vi "Get DVR From Class.vi"(8 "error in (no error)":errorcluster, 10 "Path In":path, 11 "TX Speed.lvclass In":refnum<class "TX Speed.lvclass">) -> (0 "error out":errorcluster, 2 "Class DVR":refnum<data-value>, 3 "TX Speed.lvclass Out":refnum<class "TX Speed.lvclass">)   [LabVIEW 2020, in "TX Speed.lvclass"]
uses:
  TX Speed.lvclass
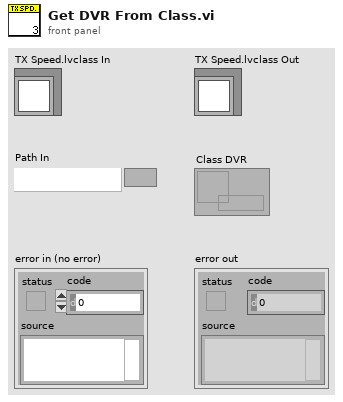
[diagram p1: front panel]
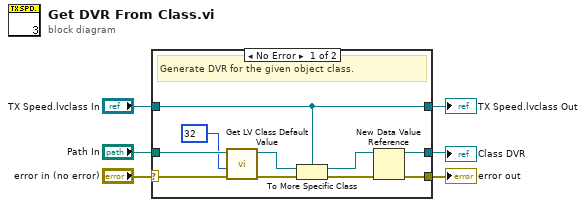
[diagram p0: block diagram]
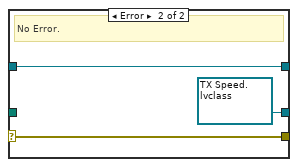
[diagram p2: hidden frame]
diagram:
  n1 = case shown="No Error" "error in (no error)" {
    selector: "error in (no error)" -> [w13 w19]
    tunnel: [w16 w19] -> w5
    tunnel: [w14 w18] -> w2
    tunnel: "TX Speed.lvclass In" -> [w14 w18]
    tunnel: "Path In" -> [w11 _]
    tunnel: [w8 refnum<data-value> refnum ("data value reference")] -> w1
    frame No Error {
      # "Generate DVR for the given object class."
      n2 = call <vilib>:"Get LV Class Default Value.vi"("error in (no error)"=w13, "options"=u32 32, "class path"=w11) -> ("error out"=w12:errorcluster, "object"=w10:refnum<class>)  [unwired: 7 in]
      n3 = To More Specific Class(target class=w14, reference=w10, error in=w12) -> (specific class reference=w9:refnum<class "TX Speed.lvclass">, error out=w15:errorcluster)
      n4 = New Data Value Reference(data value=w9, error in=w15) -> (data value reference=w8:refnum<data-value>, error out=w16:errorcluster)
    }
    frame Error {
      # "No Error."
    }
  }
  "Class DVR" <- w1
  "error out" <- w5
  "TX Speed.lvclass Out" <- w2
